vi "Get UA Variant Value.vi"(8 "error in (no error)":errorcluster, 10 "Item Id In":string, 11 "OPC UA server refnum in":T1) -> (0 "error out":errorcluster, 1 "timestamp out":timestamp, 2 "Variant Out":variant, 3 "OPC UA server refnum out":T1)   [LabVIEW 2024, in "OPCUA.lvlib"]
uses:
  <vilib>/OPCUA/controls/OPC UA Server Refnum.ctl
  <vilib>/OPCUA/server/Read Variant.vi
  OPCUA.lvlib
  <vilib>/OPCUA/NI OPC UA Server.lvlib
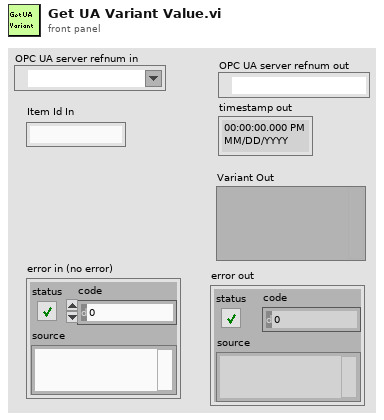
[diagram p1: front panel]
types:
  T1 = typedef "OPC UA Server Refnum.ctl" = refnum<k21>
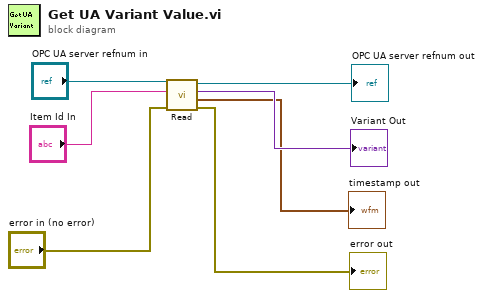
[diagram p0: block diagram]
diagram:
  n1 = call-poly <vilib>:"Read.vi"("error in (no error)"="error in (no error)", "node ID"="Item Id In", "OPC UA server refnum in"="OPC UA server refnum in") -> ("error out"=→"error out":errorcluster, "timestamp"=→"timestamp out":timestamp, "value"=→"Variant Out":variant, "OPC UA server refnum out"=→"OPC UA server refnum out":T1)  [unwired: 4 in, 1 out]
